vi "instance count allowed.vi"(8 "error in":errorcluster, 11 "Shared Library Module configuration in":refnum<class "Shared Library Module configuration.lvclass">) -> (0 "error out":errorcluster, 2 "instances allowed":i32, 3 "Shared Library Module configuration out":refnum<class "Shared Library Module configuration.lvclass">)   [LabVIEW 2013, in "Shared Library Module configuration.lvclass"]
doc: "Platypus Framework 1.0.1.60\nNI Systems Engineering - National Instruments"
uses:
  Shared Library Module configuration.lvclass
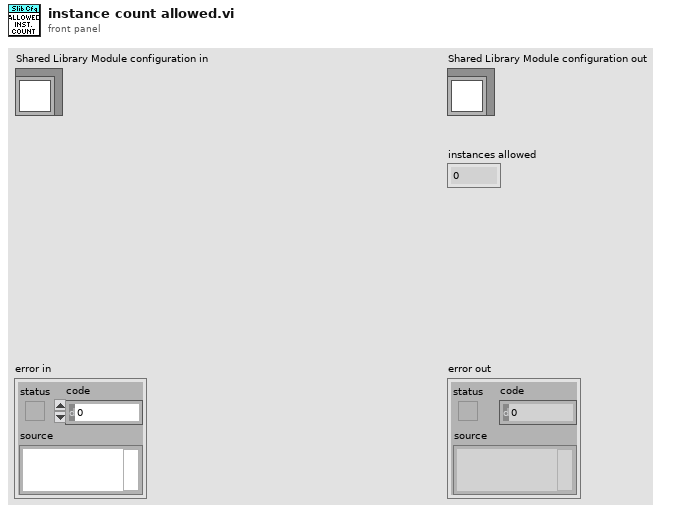
[diagram p1: front panel]
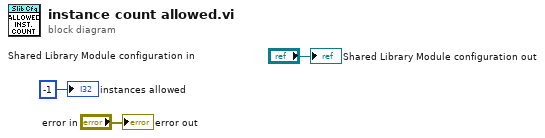
[diagram p0: block diagram]
diagram:
  "error out" <- "error in"
  "Shared Library Module configuration out" <- "Shared Library Module configuration in"
  "instances allowed" <- -1 ("instances allowed")
